vi "find index of the image name.vi"(8 "error in (no error)":errorcluster, 11 "Channel in":refnum<class "Channel.lvclass">) -> (0 "error out":errorcluster, 3 "Channel out":refnum<class "Channel.lvclass">)   [LabVIEW 2018, in "Channel.lvclass"]
uses:
  Channel.lvclass
  Channel.lvclass/Channel.ctl
  Simulated_CCD_Camera/Simulated_CCD_Camera.lvclass
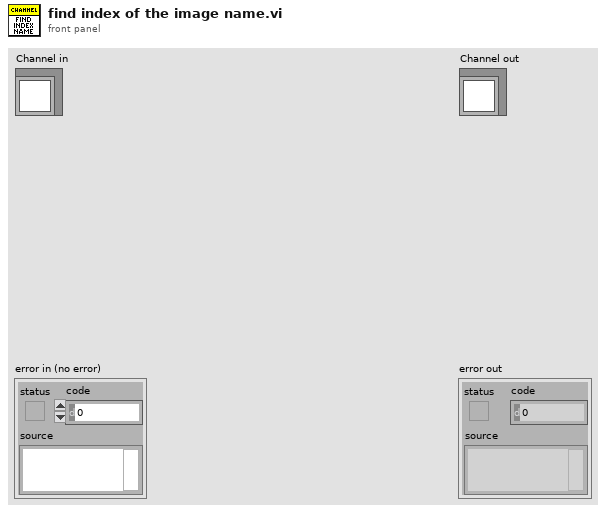
[diagram p1: front panel]
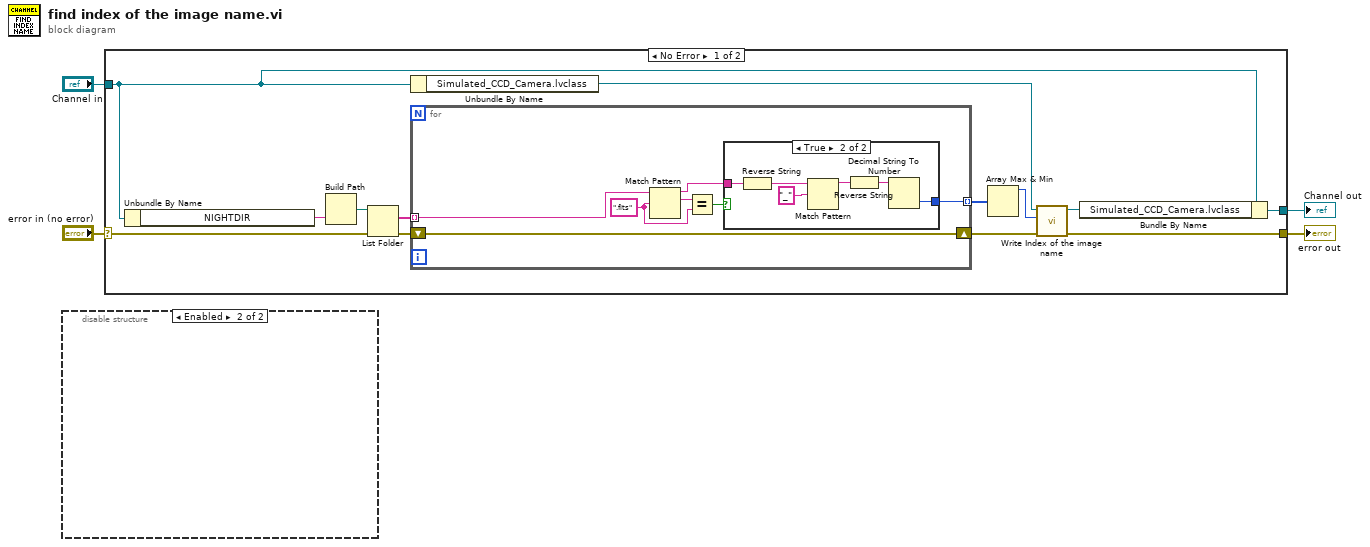
[diagram p0: block diagram]
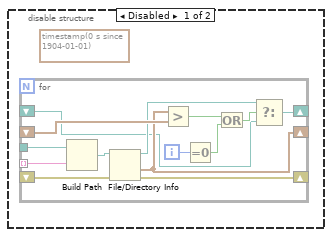
[diagram p2: hidden frame]
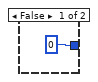
[diagram p3: hidden frame]
diagram:
  n1 = disable-structure shown="Enabled" {
    frame Disabled {
      (unwired) timestamp(0 s since 1904-01-01) ("last mod 2")
      n2 = for {
        shift-right: [w13] -> _
        shift-left: _ -> [w14]
        shift-right: [w5] -> _
        shift-left: _ -> [w6]
        shift-right: [w11] -> _
        shift-left: _ -> [w18]
        tunnel: _ -> [w10] mode=indexing
        tunnel: _ -> [w9]
        i -> [w15]
        n3 = Build Path(base path=w9, name or relative path=w10) -> (appended path=w12:path)
        n4 = File/Directory Info(path=w12, error in=w18) -> (path out=w7:path, last mod=w13:timestamp, error out=w11:errorcluster)  [unwired: 4 out]
        n5 = Greater?(x=w13, y=w14) -> (0:w17:bool)
        n6 = Equal To 0?(x=w15) -> (x = 0?=w16:bool)
        n7 = Or(x=w17, y=w16) -> (x .or. y?=w8:bool)
        n8 = Select(t=w7, s=w8, f=w6) -> (s? t:f=w5:path)
      }
    }
    frame Enabled {
    }
  }
  n9 = case shown="No Error" "error in (no error)" {
    selector: "error in (no error)" -> [w30 w47]
    tunnel: [w23 w47] -> w3
    tunnel: [w27 w46] -> w1
    tunnel: "Channel in" -> [w26 w46]
    frame No Error {
      n10 = Unbundle By Name(w26) -> ("NIGHTDIR"=w19:string)
      n11 = Build Path(name or relative path=w19) -> (appended path=w31:path)  [unwired: 1 in]
      n12 = List Folder(path=w31, error in=w30) -> (filenames=w28:string[], error out=w29:errorcluster)  [unwired: 2 in, 2 out]
      n13 = Unbundle By Name(w26) -> ("Simulated_CCD_Camera.lvclass"=w25:refnum<class "Simulated_CCD_Camera.lvclass">)
      n14 = for {
        shift-right: [w38] -> w22
        shift-left: w29 -> [w38]
        tunnel: w28 -> [w35] mode=indexing
        tunnel: [w36] -> w21 mode=indexing
        w33 = ".fits" ("regular expression")
        n15 = Match Pattern(string=w35, regular expression=w33) -> (before substring=w37:string, match substring=w34:string)  [unwired: 1 in, 2 out]
        n16 = Equal?(x=w34, y=w33) -> (x = y?=w32:bool)
        n17 = case shown="True" w32 {
          tunnel: w37 -> [_ w44]
          tunnel: [0 w40] -> w36
          frame False {
          }
          frame True {
            n18 = Reverse String(1:w44) -> (0:w43:string)
            n19 = Match Pattern(string=w43, regular expression="_") -> (before substring=w42:string)  [unwired: 1 in, 3 out]
            n20 = Reverse String(1:w42) -> (0:w45:string)
            n21 = Decimal String To Number(string=w45) -> (number=w40:i32)  [unwired: 2 in, 1 out]
          }
        }
      }
      n22 = Array Max & Min(array=w21) -> (max value=w20:i32)  [unwired: 3 out]
      n23 = call-dynamic "Write Index of the image name.vi"("error in (no error)"=w22, "Index of the image name"=w20, "Simulated_CCD_Camera in"=w25) -> ("error out"=w23:errorcluster, "Simulated_CCD_Camera out"=w24:refnum<class "Simulated_CCD_Camera.lvclass">)  [unwired: 7 in]
      n24 = Bundle By Name(cluster=w26, "Simulated_CCD_Camera.lvclass"=w24) -> (w27:refnum<class "Channel.lvclass">)
    }
    frame Error {
    }
  }
  "error out" <- w3
  "Channel out" <- w1
